vi "Actuator Control.vi"(8 "setpoint":dbl=0.6059999999999998 format="%.2f", 10 "Pot Right":T1={"DevStatus"={"status"=FALSE, "code"=0, "source"=""}, "Analog Channel"=enum."AI 1", "Invert Output"=FALSE}, 11 "Actuator Right":T3={"DeviceStatus"={"status"=FALSE, "code"=0, "source"=""}, "Type"=enum."CAN", "PWM"={"PWM Channel"=enum."PWM 1", "DeadBand"={"Name"="", "maxPositivePwm"=0, "minPositivePwm"=0, "centerPwm"=0, "maxNegativePwm"=0, "minNegativePwm"=0, "angularRange"=0}}, "CAN"={"Device Number"=5, "SetOutput VI Ref"=variant(refnum<vi> refnum), "GetOutput VI Ref"=variant(refnum<vi> refnum), "Enable VI Ref"=variant(refnum<vi> refnum), "Disable VI Ref"=variant(refnum<vi> refnum), "Data"=variant(cluster{"Library":path, "handle":u64, "Control Mode":u16, "UsageFrame":u32, "RefNumName":string, "arbID":u32} {"Library"=path "libCTRE_PhoenixCCI.so", "handle"=38440496, "Control Mode"=0, "UsageFrame"=0, "RefNumName"="", "arbID"=33816581})}, "Invert"=FALSE, "DIO PWM"={"PWM \"Enable\" Channel"=enum."Invalid", "DIOChannel"=enum."Invalid", "PWM Rate"=0.0}}) -> ()   [LabVIEW 2017]
uses:
  <vilib>/Rock Robotics/WPI/MotorControl/WPI_MotorControlDeviceRef.ctl
  <vilib>/Rock Robotics/WPI/MotorControl/WPI_MotorControlType.ctl
  <vilib>/Rock Robotics/SystemInterfaces/DIO/FPGA_DIOPWMChannel.ctl
  <vilib>/Rock Robotics/WPI/PWM/WPI_PWMDeadband.ctl
  <vilib>/Rock Robotics/SystemInterfaces/DIO/FPGA_DIOChannel.ctl
  <vilib>/Rock Robotics/WPI/Potentiometer/WPI_PotentiometerDevRef.ctl
  <vilib>/Rock Robotics/SystemInterfaces/AI/FPGA_AIChannel.ctl
panel:
  in  "Accepted Range":dbl=0.009000000000000001 format="%#_13g"
  in  "p":dbl=1.0
  in  "subraction":dbl=-0.05
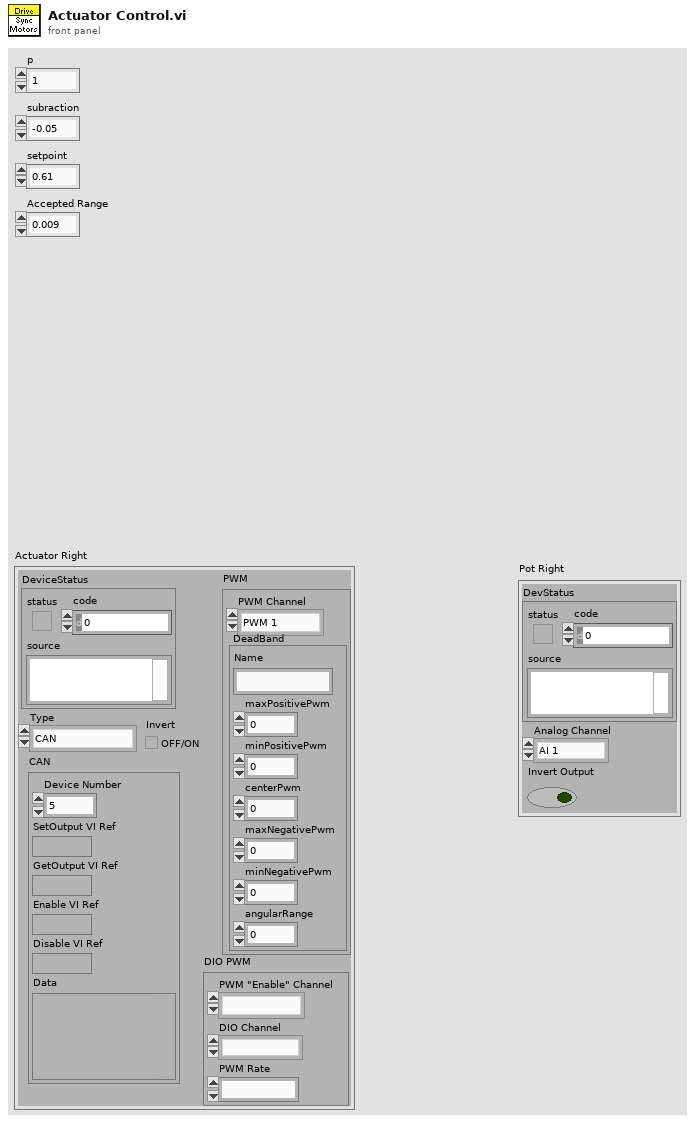
[diagram p1: front panel]
types:
  T1 = typedef "WPI_PotentiometerDevRef.ctl" = cluster{"DevStatus":errorcluster, "Analog Channel":T2, "Invert Output":bool}
  T2 = typedef "FPGA_AIChannel.ctl" = enum8{"AI 0", "AI 1", "AI 2", "AI 3", "AI MXP 0", "AI MXP 1", "AI MXP 2", "AI MXP 3", "Invalid"}
  T3 = typedef "WPI_MotorControlDeviceRef.ctl" = cluster{"DeviceStatus":errorcluster, "Type":T4, "PWM":cluster{"PWM Channel":T5, "DeadBand":T6}, "CAN":cluster{"Device Number":u8, "SetOutput VI Ref":variant, "GetOutput VI Ref":variant, "Enable VI Ref":variant, "Disable VI Ref":variant, "Data":variant}, "Invert":bool, "DIO PWM":cluster{"PWM \"Enable\" Channel":T5, "DIOChannel":T7, "PWM Rate":dbl}}
  T4 = typedef "WPI_MotorControlType.ctl" = enum16{"PWM", "CAN", "DIO PWM"}
  T5 = typedef "FPGA_DIOPWMChannel.ctl" = enum8{"PWM 0", "PWM 1", "PWM 2", "PWM 3", "PWM 4", "PWM 5", "PWM 6", "PWM 7", "PWM 8", "PWM 9", "PWM MXP 0", "PWM MXP 1", "PWM MXP 2", "PWM MXP 3", "PWM MXP 4", "PWM MXP 5", "PWM MXP 6", "PWM MXP 7", "PWM MXP 8", "PWM MXP 9", "Invalid"}
  T6 = typedef "WPI_PWMDeadband.ctl" = cluster{"Name":string, "maxPositivePwm":i32, "minPositivePwm":i32, "centerPwm":i32, "maxNegativePwm":i32, "minNegativePwm":i32, "angularRange":u16}
  T7 = typedef "FPGA_DIOChannel.ctl" = enum8{"DIO 0", "DIO 1", "DIO 2", "DIO 3", "DIO 4", "DIO 5", "DIO 6", "DIO 7", "DIO 8", "DIO 9", "DIO MXP 0", "DIO MXP 1", "DIO MXP 2", "DIO MXP 3", "DIO MXP 4", "DIO MXP 5", "DIO MXP 6", "DIO MXP 7", "DIO MXP 8", "DIO MXP 9", "DIO MXP 10", "DIO MXP 11", "DIO MXP 12", "DIO MXP 13", "DIO MXP 14", "DIO MXP 15", "SPI Port CS1", "SPI Port CS2", "SPI Port CS3", "SPI Port MISO", "SPI Port MOSI", "Invalid"}
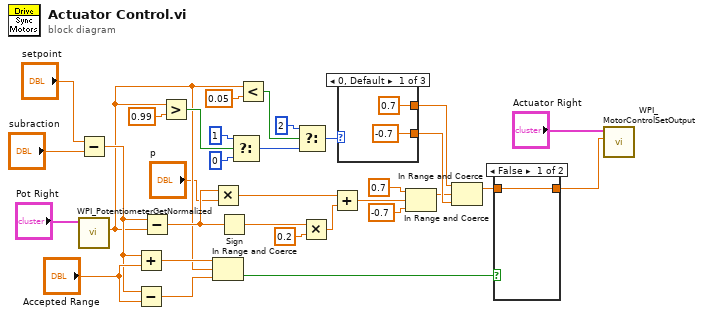
[diagram p0: block diagram]
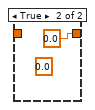
[diagram p2: hidden frame]
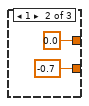
[diagram p3: hidden frame]
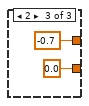
[diagram p4: hidden frame]
diagram:
  n1 = Subtract(x="setpoint", y="subraction") -> (x-y=w6:dbl)
  n2 = call <vilib>:"WPI_PotentiometerGetNormalized.vi"("PotDevRef"="Pot Right") -> ("Normalized Value"=w3:dbl)  [unwired: 8 in, 2 out]
  n3 = Add(x=w6, y="Accepted Range") -> (x+y=w11:dbl)
  n4 = Subtract(x=w6, y="Accepted Range") -> (x-y=w10:dbl)
  n5 = Subtract(x=w6, y=w3) -> (x-y=w17:dbl)
  n6 = Greater?(x=w3, y=0.99) -> (0:w19:bool)
  n7 = Multiply(x=w17, y="p") -> (x*y=w2:dbl)
  n8 = In Range and Coerce(upper limit=w11, x=w3, lower limit=w10) -> (In Range?=w9:bool)  [unwired: 1 out]
  n9 = Sign(1:w17) -> (0:w16:dbl)
  n10 = Select(t=u32 1, s=w19, f=u32 0) -> (s? t:f=w24:u32)
  n11 = Less?(x=w3, y=0.05) -> (x < y?=w20:bool)
  n12 = Select(t=u32 2, s=w20, f=w24) -> (s? t:f=w26:u32)
  n13 = Multiply(x=w16, y=0.2) -> (x*y=w15:dbl)
  n14 = Add(x=w2, y=w15) -> (x+y=w14:dbl)
  n15 = case shown="0, Default" w26 {
    tunnel: [0.7 ("upper limit") 0.0 ("upper limit") -0.7 ("upper limit")] -> w23
    tunnel: [-0.7 ("upper limit") -0.7 ("upper limit") 0.0 ("upper limit")] -> w22
    frame 0, Default {
    }
    frame 1 {
    }
    frame 2 {
    }
  }
  n16 = In Range and Coerce(upper limit=0.7, x=w14, lower limit=-0.7) -> (coerced(x)=w21:dbl)  [unwired: 1 out]
  n17 = In Range and Coerce(upper limit=w23, x=w21, lower limit=w22) -> (coerced(x)=w8:dbl)  [unwired: 1 out]
  n18 = case shown="False" w9 {
    tunnel: w8 -> [w40 _]
    tunnel: [w40 0.0 ("upper limit")] -> w7
    frame False {
    }
    frame True {
      (unwired) 0.0 ("upper limit")
    }
  }
  n19 = call <vilib>:"WPI_MotorControlSetOutput.vi"("Output"=w7, "MotorControlDevRef"="Actuator Right") -> ()  [unwired: 7 in, 3 out]
